vi "UMB_IR_WallAvoid.vi"(8 "behavior weights":i8[](array[numeric]), 10 "tweak cluster":T1={"Lider good scale mult"=0.0, "Lider good scale add"=0.0, "Lider speed scale mult"=0.0, "Lider speed scale add"=0.0, "Follow right?"=FALSE, "IR Following Distance"=400, "IR scaling div"=0.0, "Numeric"=0.0}, 11 "ir distance":i32) -> (3 "Behavior Output":T2)   [LabVIEW 2012]
uses:
  NINJA Code/Tugboat/Robo_Programs/behaviorOutput_t.ctl
  <vilib>/gmath/statdist.llb/Normal PDF.vi
  <vilib>/gmath/NI_Gmath.lvlib
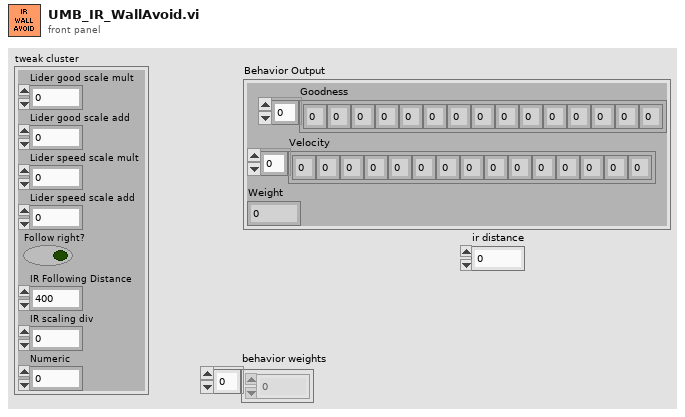
[diagram p1: front panel]
types:
  T1 = cluster{"Lider good scale mult":dbl, "Lider good scale add":dbl, "Lider speed scale mult":dbl, "Lider speed scale add":dbl, "Follow right?":bool, "IR Following Distance":i32, "IR scaling div":dbl, "Numeric":dbl}
  T2 = typedef "behaviorOutput_t.ctl" = cluster{"Goodness":i8[], "Velocity":i8[], "Weight":i8}
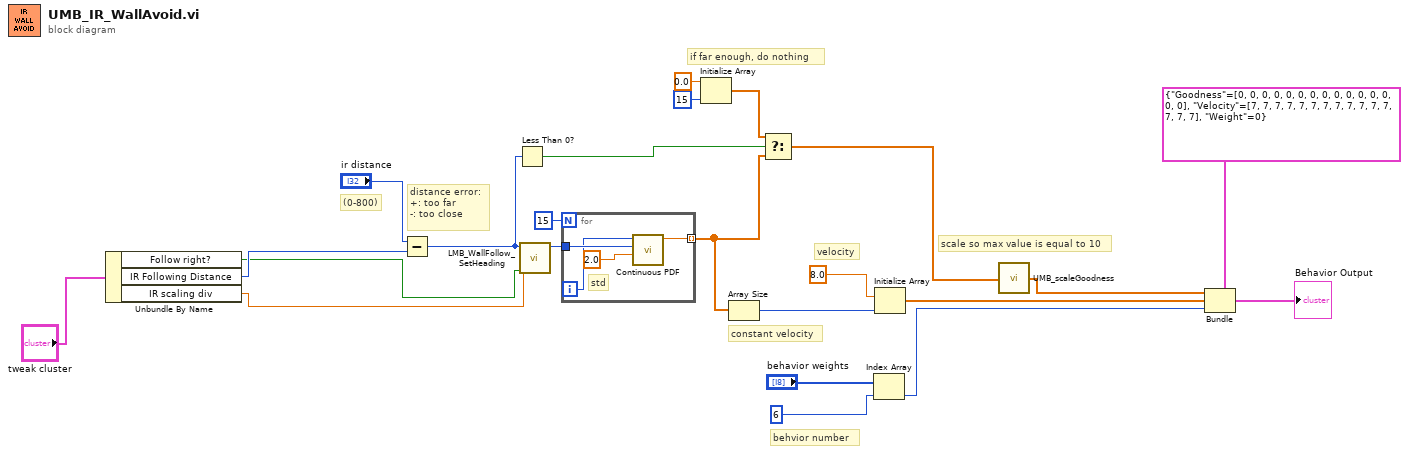
[diagram p0: block diagram]
diagram:
  # "if far enough, do nothing"
  # "scale so max value is equal to 10"
  # "(0-800)"
  # "constant velocity"
  # "velocity"
  # "distance error: \n+: too far\n-: too close"
  # "behvior number"
  n1 = Unbundle By Name("tweak cluster") -> ("Follow right?"=w10:bool, "IR Following Distance"=w11:i32, "IR scaling div"=w12:dbl)
  n2 = Subtract(x="ir distance", y=w11) -> (x-y=w7:i32)
  n3 = Less Than 0?(x=w7) -> (x < 0?=w1:bool)
  n4 = call "LMB_WallFollow_SetHeading.vi"("Follow Right?"=w10, "division constant"=w12, "Distance error"=w7) -> ("heading"=w17:i32)  [unwired: 8 in]
  n5 = for {
    N: 15 -> [_]
    tunnel: w17 -> [w27]
    tunnel: [w25] -> w3 mode=indexing
    i -> [w24]
    # "std"
    n6 = call-poly <vilib>:"Continuous PDF.vi"("std"=2.0, "mean"=w27, "x"=w24) -> ("pdf(x)"=w25:dbl)  [unwired: 7 in, 1 out]
  }
  n7 = Initialize Array(0.0 ("element"), 15 ("dimension size")) -> (w2:dbl[])
  n8 = Array Size(array=w3) -> (size(s)=w14:i32)
  n9 = Select(t=w2, s=w1, f=w3) -> (s? t:f=w4:dbl[])
  n10 = Index Array(array="behavior weights", index=6) -> (element=w21:i8)
  n11 = Initialize Array(8.0 ("element"), w14) -> (w15:dbl[])
  n12 = call "UMB_scaleGoodness.vi"("goodness"=w4) -> ("scaled goodness"=w8:dbl[])
  n13 = Bundle(cluster=T2 {"Goodness"=[0, 0, 0, 0, 0, 0, 0, 0, 0, 0, 0, 0, 0, 0, 0], "Velocity"=[7, 7, 7, 7, 7, 7, 7, 7, 7, 7, 7, 7, 7, 7, 7], "Weight"=0} ("Behavior Output"), "Goodness"=w8, "Velocity"=w15, "Weight"=w21) -> (→"Behavior Output":T2)
